vi "Conditionally Create Default Terminal Name.vi"(8 "error in":errorcluster, 10 "terminal address in":T1, 11 "terminal name in":string) -> (0 "error out":errorcluster, 3 "terminal name out":string)   [LabVIEW 2020, in "Ballard MIL-STD-1553 Scripting.lvlib"]
uses:
  Ballard MIL-STD-1553 Scripting.lvlib
  Constants.vi
  Shared/Address.ctl
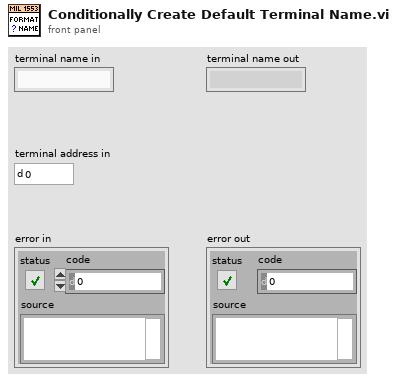
[diagram p1: front panel]
types:
  T1 = typedef "Address.ctl" = u16
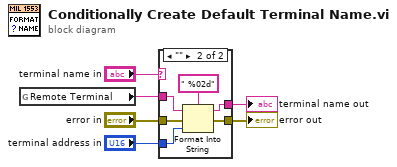
[diagram p0: block diagram]
diagram:
  n1 = global read "Constants.vi" "Remote Terminal"() -> (w4:string)
  n2 = case shown="\"\"" "terminal name in" {
    selector: "terminal name in" -> [w8 _]
    tunnel: "error in" -> [w7 w13]
    tunnel: [w7 w12] -> w2
    tunnel: "terminal address in" -> [_ w9]
    tunnel: w4 -> [_ w11]
    tunnel: [w8 w10] -> w6
    frame Default {
    }
    frame "" {
      n3 = Format Into String(format string=" %02d", initial string=w11, error in=w13, w9) -> (resulting string=w10:string, error out=w12:errorcluster)
    }
  }
  "terminal name out" <- w6
  "error out" <- w2
